vi "Add to Most Recent Used List.vi"(8 "错误输入（无错误）":errorcluster, 11 "Path":path) -> (0 "错误输出":errorcluster)   [LabVIEW 2012, in "Application.lvlib"]
uses:
  Application.lvlib
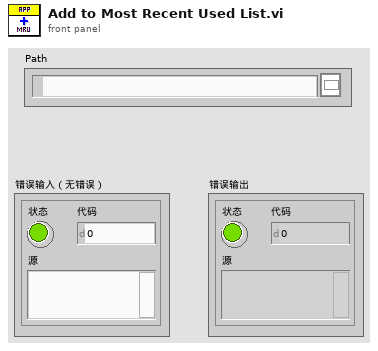
[diagram p1: front panel]
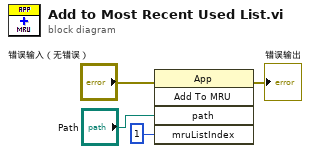
[diagram p0: block diagram]
diagram:
  n1 = invoke class="App" method="Add To MRU"(error in="错误输入（无错误）", "path"="Path", "mruListIndex"=1 ("Most Recently Used List Index")) -> (error out=→"错误输出":errorcluster)  [unwired: 2 in, 4 out]
